vi "GF_StartShotLog.vi"(2 "error in":errorcluster, 3 "Shot Number":i32, 4 "Shot Notes":string) -> (0 "error out":errorcluster, 1 "Shotlog Beginning":string)   [LabVIEW 2009]
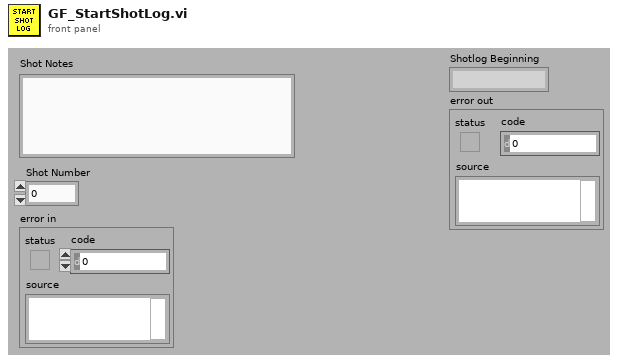
[diagram p1: front panel]
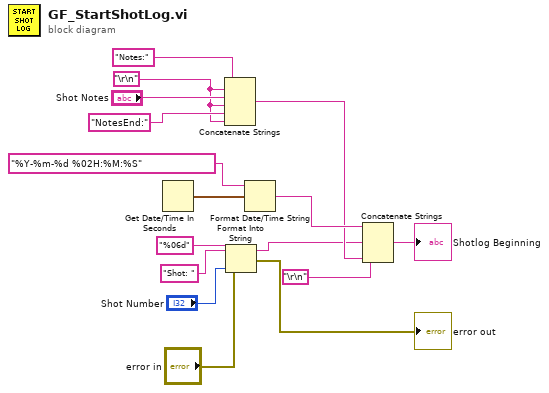
[diagram p0: block diagram]
diagram:
  w9 = "\r\n"
  w13 = "\r\n"
  n1 = Get Date/Time In Seconds() -> (seconds since 1Jan1904=w14:timestamp)
  n2 = Concatenate Strings("Notes:" ("string"), w9, "Shot Notes", w9, "NotesEnd:" ("string"), w9) -> (w8:string)
  n3 = Format Into String(format string="%06d", initial string="Shot: ", error in="error in", "Shot Number") -> (resulting string=w6:string, error out=→"error out":errorcluster)
  n4 = Format Date/Time String(time format string (%c)="%Y-%m-%d %02H:%M:%S", seconds (now)=w14) -> (date/time string=w15:string)  [unwired: 1 in]
  n5 = Concatenate Strings(w15, w13, w6, w13, w8) -> (→"Shotlog Beginning":string)
